vi "Wait for Acquisition Complete.vi"(8 "error in (no error)":errorcluster, 10 "Maximum Time (10000 ms)":i32=10000, 11 "VISA resource name":refnum<visa-resource-name>) -> (0 "error out":errorcluster, 3 "VISA resource name out":refnum<visa-resource-name>)   [LabVIEW 2022 SP3, in "Agilent N934X Series.lvlib"]
doc: "Waits for the current sweep to finish. You can use this VI after Initiate VI and before Fetch Trace VI.\n\nNote:\n\nThis VI does not check the instrument status. Typically, you call this VI only in a sequence of calls to other low-level instrument driver VIs. The sequence performs one operation. You use the low-level VIs to optimize one or more aspects of interaction with the instrument. If you want to check the instrument status, call the <B>Error Query VI</B> at the conclusion of the sequence."
uses:
  <instrlib>/Agilent N934X Series/Agilent N934X Series.lvlib
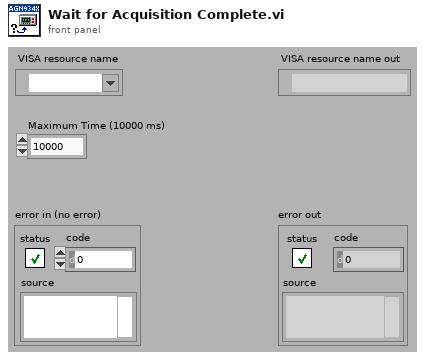
[diagram p1: front panel]
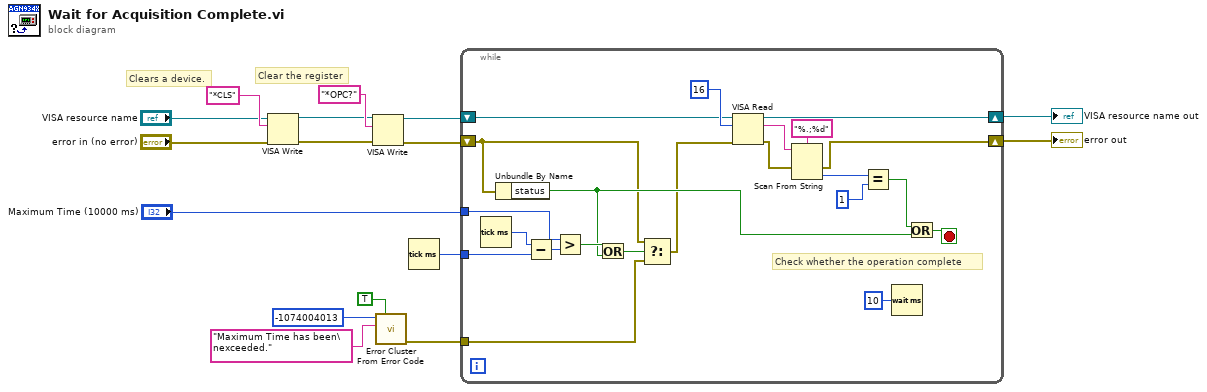
[diagram p0: block diagram]
diagram:
  # "Clears a device."
  # "Clear the register"
  n1 = VISA Write(VISA resource name="VISA resource name", write buffer="*CLS", error in (no error)="error in (no error)") -> (VISA resource name out=w10:refnum<visa-resource-name>, error out=w9:errorcluster)  [unwired: 1 out]
  n2 = VISA Write(VISA resource name=w10, write buffer="*OPC?", error in (no error)=w9) -> (VISA resource name out=w7:refnum<visa-resource-name>, error out=w8:errorcluster)  [unwired: 1 out]
  n3 = call <vilib>:"Error Cluster From Error Code.vi"("show call chain? (False)"=TRUE, "error message (\"\")"="Maximum Time has been\nexceeded." ("error message (\"\")"), "error code (0)"=-1074004013) -> ("error out"=w12:errorcluster)  [unwired: 1 in, 5 out]
  n4 = Tick Count (ms)() -> (millisecond timer value=w16:u32)
  n5 = while {
    tunnel: "Maximum Time (10000 ms)" -> [w29]
    tunnel: w16 -> [w33]
    tunnel: w12 -> [w24]
    shift-right: [w31] -> w4
    shift-left: w8 -> [w23]
    shift-right: [w36] -> w5
    shift-left: w7 -> [w20]
    stop <- w30 stop-if-true
    # "Check whether the operation complete"
    n6 = Tick Count (ms)() -> (millisecond timer value=w34:u32)
    n7 = Unbundle By Name(w23) -> ("status"=w25:bool)
    n8 = Subtract(x=w34, y=w33) -> (x-y=w28:u32)
    n9 = Greater?(x=w29, y=w28) -> (0:w27:bool)
    n10 = Or(x=w27, y=w25) -> (x .or. y?=w26:bool)
    n11 = Select(t=w23, s=w26, f=w24) -> (s? t:f=w21:errorcluster)
    n12 = VISA Read(VISA resource name=w20, byte count=u32 16, error in (no error)=w21) -> (VISA resource name out=w36:refnum<visa-resource-name>, read buffer=w38:string, error out=w32:errorcluster)  [unwired: 1 out]
    n13 = Scan From String(format string="%.;%d", input string=w38, error in=w32) -> (error out=w31:errorcluster, output 1=w19:i32)  [unwired: 1 in, 3 out]
    n14 = Equal?(x=w19, y=1 ("index")) -> (x = y?=w17:bool)
    n15 = Wait (ms)(milliseconds to wait=u32 10) -> ()  [unwired: 1 out]
    n16 = Or(x=w17, y=w25) -> (x .or. y?=w30:bool)
  }
  "error out" <- w4
  "VISA resource name out" <- w5
